vi "SPI Block Read Bytes Of Event.vi"(1 "TimeOutOfMs":i32, 4 "EventType":u8, 5 "EventPin":i32, 6 "BlockNum":i32, 7 "BlockSize":i32, 9 "pReadData":u8[](array[numeric])=array[4097 elements], 10 "SPIIndex":i32, 11 "DevHandle":i32) -> (2 "function return":i32, 3 "pReadData out":u8[](array[numeric]))   [LabVIEW 2010, in "usb2spi.lvlib"]
doc: "int WINAPI SPI_BlockReadBytesOfEvent(int DevHandle,int SPIIndex,unsigned char *pReadData,int BlockSize,int BlockNum,int EventPin,unsigned char EventType,int TimeOutOfMs);"
uses:
  usb2spi.lvlib
  USB2XXX/trunk/USB2XXX/USB2XXX/vs2019/Release/USB2XXX.dll
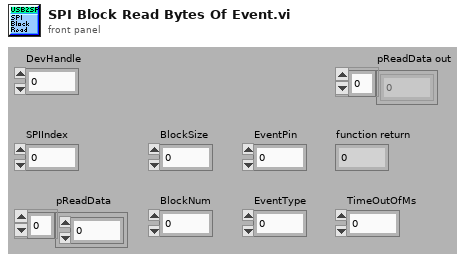
[diagram p1: front panel]
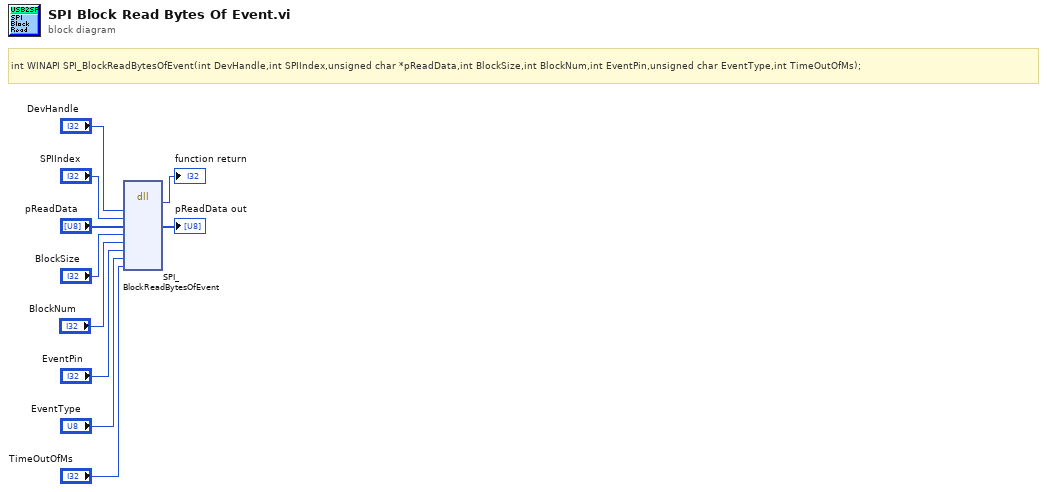
[diagram p0: block diagram]
diagram:
  # "int WINAPI SPI_BlockReadBytesOfEvent(int DevHandle,int SPIIndex,unsigned char *pReadData,int BlockSize,int BlockNum,int EventPin,unsigned char EventType,int TimeOutOfMs);"
  n1 = dll-call lib="E:/Projects/USB2XXX/trunk/USB2XXX/USB2XXX/vs2019/Release/USB2XXX.*" fn="SPI_BlockReadBytesOfEvent"("DevHandle"="DevHandle", "SPIIndex"="SPIIndex", "pReadData"="pReadData", "BlockSize"="BlockSize", "BlockNum"="BlockNum", "EventPin"="EventPin", "EventType"="EventType", "TimeOutOfMs"="TimeOutOfMs") -> (→"function return":i32, "pReadData"=→"pReadData out":u8[])  [unwired: 10 in, 2 out]
